vi "poly_h5_append_array_1d_to_2d.vi"(8 "error in":errorcluster, 9 "dim (1)":enum16{"1", "2"}(ring), 10 "1d array":dbl[](array[numeric]), 11 "h5 2d array ref":T1 format="%.0x") -> (0 "error out":errorcluster)   [LabVIEW 2015]
uses:
  <vilib>/addons/h5labview2/base/hid_t.ctl
  <vilib>/addons/h5labview2/base/lib_path.vi
  <vilib>/addons/h5labview2/base/H5Equery.vi
  <vilib>/addons/h5labview2/dataset/H5Dwrite.llb/H5Dwrite.xnode
  <vilib>/addons/h5labview2/dataset/H5D.lvlib
  <vilib>/addons/h5labview2/space/H5S.lvlib
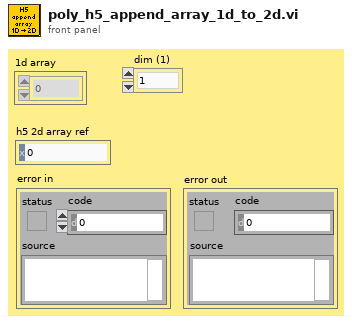
[diagram p1: front panel]
types:
  T1 = typedef "hid_t.ctl" = i32
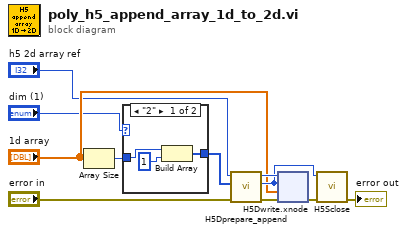
[diagram p0: block diagram]
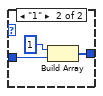
[diagram p2: hidden frame]
diagram:
  n1 = Array Size(array="1d array") -> (size(s)=w6:i32)
  n2 = case shown="\"2\"" "dim (1)" {
    tunnel: w6 -> [w13 w16]
    tunnel: [w12 w15] -> w5
    frame "2" {
      n3 = Build Array(w13, 1 ("ndims")) -> (w12:i32[])
    }
    frame "1" {
      n4 = Build Array(1 ("ndims"), w16) -> (w15:i32[])
    }
  }
  n5 = call <vilib>:"H5Dprepare_append.vi"("error in (no error)"="error in", "append dims"=w5, "dset in"="h5 2d array ref") -> ("error out"=w9:errorcluster, "space out"=w10:T1, "dset out"=w11:T1)  [unwired: 5 in, 1 out]
  n6 = xnode "H5Dwrite.xnode"("error in (no error)"=w9, "data"="1d array", "file space"=w10, "ref in"=w11) -> ("error out"=w8:errorcluster)  [unwired: 3 in, 2 out]
  n7 = call <vilib>:"H5Sclose.vi"("error in (no error)"=w8, "space in"=w10) -> ("error out"=→"error out":errorcluster)  [unwired: 9 in]
